vi "SetPincherState.vi"(8 "error in":errorcluster, 11 "PincherState":enum16{"Open", "Close"}(ring)) -> (0 "error out":errorcluster)   [LabVIEW 2016]
doc: "Sets pincher state global variable"
uses:
  Robot Global Data.vi
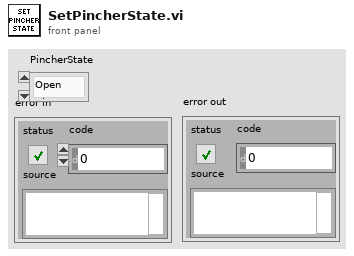
[diagram p1: front panel]
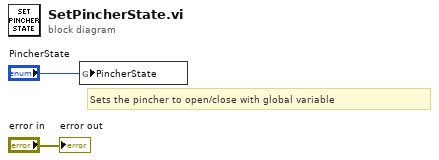
[diagram p0: block diagram]
diagram:
  # "Sets the pincher to open/close with global variable"
  n1 = global write "Robot Global Data.vi" "PincherState"("PincherState") -> ()
  "error out" <- "error in"
